vi "VI Tree.vi"   [LabVIEW 2020, in "Agilent 34401.lvlib"]
doc: "This is the instrument driver for the Keysight/Agilent 34401A, 34410A, 34411A, L4411A digital multimeters."
uses:
  <instrlib>/Agilent 34401/Agilent 34401.lvlib
  <instrlib>/Agilent 34401/Public/Data/Read (Math).vi
  <instrlib>/Agilent 34401/Public/Configure/Configure Temperature (RTD).vi
  <instrlib>/Agilent 34401/Public/Data/Read (Transient).vi
  <instrlib>/Agilent 34401/Public/Data/Read (Multiple Points).vi
  <instrlib>/Agilent 34401/Public/Data/Read (Single Point).vi
panel:
  # "(c) 2005-2015 National Instruments.  ALL RIGHTS RESERVED."
  # "SEE DIAGRAM\nFOR VI Tree"
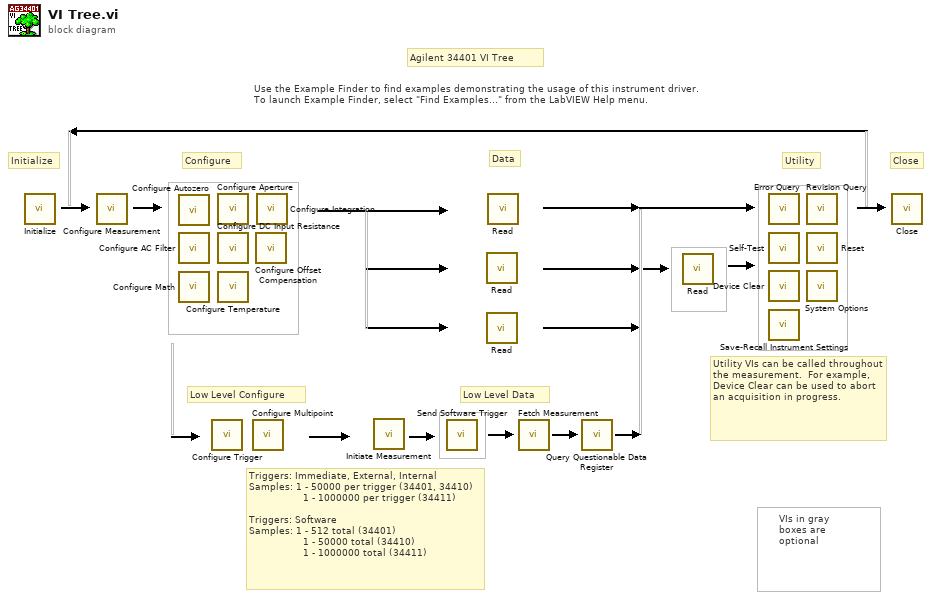
[diagram p0: block diagram]
diagram:
  # "Utility VIs can be called throughout the measurement.  For example, Device Clear can be used to abort an acquisition in progress."
  # "Use the Example Finder to find examples demonstrating the usage of this instrument driver.\nTo launch Example Finder, select \"Find Examples...\" from the LabVIEW Help menu."
  # "Triggers: Immediate, External, Internal\nSamples: 1 - 50000 per trigger (34401, 34410)\n                  1 - 1000000 per trigger (34411)\n\nTriggers: Software\nSamples: 1 - 512 total (34401)\n                  1 - 50000 total (34410)\n                  1 - 1000000 total (34411)"
  # "VIs in gray\nboxes are\noptional"
  # "Agilent 34401 VI Tree"
  # "Low Level Configure"
  # "Low Level Data"
  # "Configure"
  # "Utility"
  # "Data"
  # "Close"
  # "Initialize"
  n1 = call <instrlib>:"Initialize.vi"() -> ()  [unwired: 10 in, 2 out]
  n2 = call <instrlib>:"Configure Measurement.vi"() -> ()  [unwired: 10 in, 2 out]
  n3 = call <instrlib>:"Configure Autozero.vi"() -> ()  [unwired: 10 in, 2 out]
  n4 = call <instrlib>:"Configure AC Filter.vi"() -> ()  [unwired: 10 in, 2 out]
  n5 = call <instrlib>:"Configure Math.vi"() -> ()  [unwired: 14 in, 2 out]
  n6 = call <instrlib>:"Configure Trigger.vi"() -> ()  [unwired: 10 in, 2 out]
  n7 = call <instrlib>:"Configure Aperture.vi"() -> ()  [unwired: 10 in, 2 out]
  n8 = call <instrlib>:"Configure DC Input Resistance.vi"() -> ()  [unwired: 10 in, 2 out]
  n9 = call-poly <instrlib>:"Configure Temperature.vi"() -> ()  [unwired: 14 in, 2 out]
  n10 = call <instrlib>:"Configure Multipoint.vi"() -> ()  [unwired: 10 in, 2 out]
  n11 = call <instrlib>:"Configure Offset Compensation.vi"() -> ()  [unwired: 10 in, 2 out]
  n12 = call <instrlib>:"Configure Integration.vi"() -> ()  [unwired: 10 in, 2 out]
  n13 = call <instrlib>:"Initiate Measurement.vi"() -> ()  [unwired: 10 in, 2 out]
  n14 = call <instrlib>:"Send Software Trigger.vi"() -> ()  [unwired: 10 in, 2 out]
  n15 = call-poly <instrlib>:"Read.vi"() -> ()  [unwired: 9 in, 3 out]
  n16 = call-poly <instrlib>:"Read.vi"() -> ()  [unwired: 6 in, 6 out]
  n17 = call-poly <instrlib>:"Read.vi"() -> ()  [unwired: 9 in, 3 out]
  n18 = call <instrlib>:"Fetch Measurement.vi"() -> ()  [unwired: 8 in, 4 out]
  n19 = call <instrlib>:"Query Questionable Data Register.vi"() -> ()  [unwired: 9 in, 3 out]
  n20 = call-poly <instrlib>:"Read.vi"() -> ()  [unwired: 4 in, 8 out]
  n21 = call <instrlib>:"Error Query.vi"() -> ()  [unwired: 8 in, 4 out]
  n22 = call <instrlib>:"Self-Test.vi"() -> ()  [unwired: 8 in, 4 out]
  n23 = call <instrlib>:"Device Clear.vi"() -> ()  [unwired: 10 in, 2 out]
  n24 = call <instrlib>:"Save-Recall Instrument Settings.vi"() -> ()  [unwired: 10 in, 2 out]
  n25 = call <instrlib>:"Revision Query.vi"() -> ()  [unwired: 8 in, 4 out]
  n26 = call <instrlib>:"Reset.vi"() -> ()  [unwired: 10 in, 2 out]
  n27 = call <instrlib>:"System Options.vi"() -> ()  [unwired: 10 in, 2 out]
  n28 = call <instrlib>:"Close.vi"() -> ()  [unwired: 11 in, 1 out]
